vi "Delete Bucket Website Configuration.vi"(4 "Region":T1, 8 "error in (no error)":errorcluster, 9 "Bucket":string) -> (0 "error out":errorcluster)   [LabVIEW 2015, in "LV Interface for Amazon S3.lvlib"]
doc: "<B>Removes</B> the <B>website configuration</B> for a bucket. This operation <B>requires</B> the <B>S3:DeleteBucketWebsite permission</B>. By default, only the bucket owner can delete the website configuration attached to a bucket. Bucket <B>owners can grant</B> other <B>users permission to delete the website configuration</B> by writing a bucket policy <B>granting them the S3:DeleteBucketWebsite permission</B>."
uses:
  LV Interface for Amazon S3.lvlib
  Typedefs/AMZ_S3_LocationConstraint.ctl
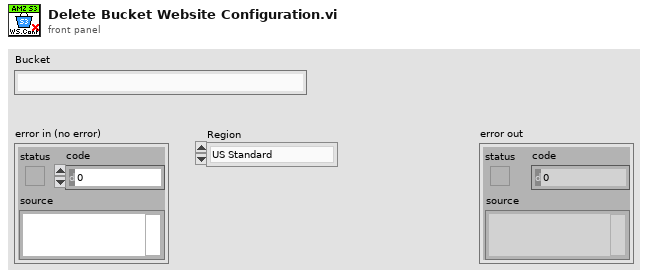
[diagram p1: front panel]
types:
  T1 = typedef "LV Interface for Amazon S3.lvlib/AMZ_S3_LocationConstraint.ctl" = enum16{"US Standard", "us-east-2", "us-west-1", "us-west-2", "ap-northeast-1", "ap-northeast-2", "ap-southeast-1", "ap-southeast-2", "ca-central-1", "eu-central-1", "eu-west-1", "eu-west-2", "sa-east-1"}
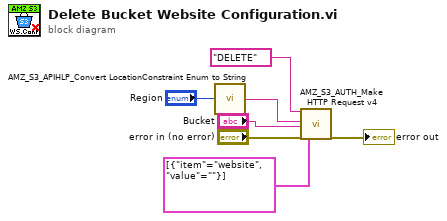
[diagram p0: block diagram]
diagram:
  n1 = call "AMZ_S3_APIHLP_Convert LocationConstraint Enum to String.vi"("Location"="Region") -> ("Location String"=w1:string)  [unwired: 4 in]
  n2 = call "AMZ_S3_AUTH_Make HTTP Request v4.vi"("HTTP-Verb"="DELETE", "Region"=w1, "Bucket"="Bucket", "error in"="error in (no error)", "request parameters"=cluster{"item":string, "value":string}[] [{"item"="website", "value"=""}]) -> ("error out"=→"error out":errorcluster)  [unwired: 11 in, 3 out]
